vi "niRFSTS SG Close.vi"(11 "TSM Context":T1) -> (0 "error out":errorcluster)   [LabVIEW 2014]
uses:
  <vilib>/NI_TestStand_SemiconductorModule/NI_TestStand_Semiconductor_Module.lvlibp/PinMap/General/SemiconductorModuleContext.ctl
  <vilib>/NI_TestStand_SemiconductorModule/NI_TestStand_Semiconductor_Module.lvlibp/PinMap/RF/RFSG/PinToNIRFSGSessions.vi
  <vilib>/NI_TestStand_SemiconductorModule/NI_TestStand_Semiconductor_Module.lvlibp
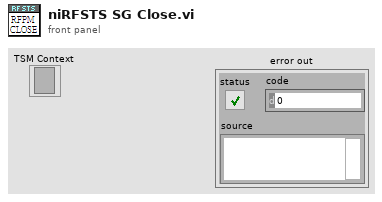
[diagram p1: front panel]
types:
  T1 = typedef "NI_TestStand_Semiconductor_Module.lvlibp/SemiconductorModuleContext.ctl" = refnum<k7>
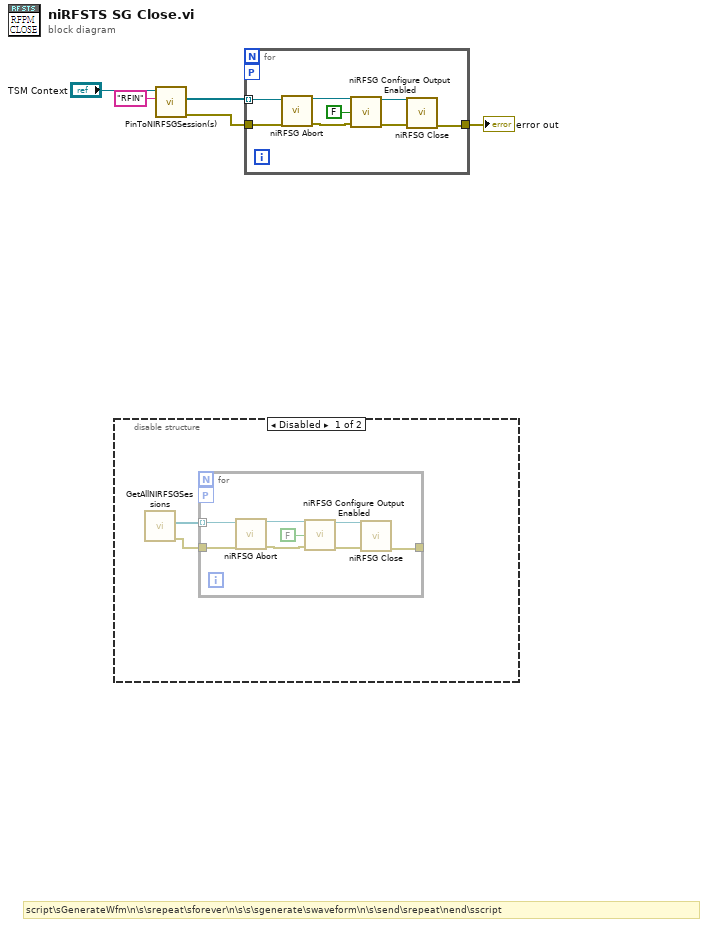
[diagram p0: block diagram]
diagram:
  # "script\\sGenerateWfm\\n\\s\\srepeat\\sforever\\n\\s\\s\\sgenerate\\swaveform\\n\\s\\send\\srepeat\\nend\\sscript"
  n1 = disable-structure shown="Disabled" {
    frame Disabled {
      n2 = call <vilib>:"GetAllNIRFSGSessions.vi"() -> ("error out"=w7:errorcluster, "Instrument Sessions"=w6:refnum<k15>[])  [unwired: 9 in, 1 out]
      n3 = for {
        workers-P: _ -> [_]
        tunnel: w6 -> [w11] mode=indexing
        tunnel: w7 -> [w10]
        tunnel: [w12] -> _
        n4 = call <instrlib>:"niRFSG Abort.vi"("instrument handle"=w11, "error in"=w10) -> ("instrument handle out"=w8:refnum<k15>, "error out"=w9:errorcluster)  [unwired: 12 in]
        n5 = call <instrlib>:"niRFSG Configure Output Enabled.vi"("instrument handle"=w8, "output enabled"=FALSE, "error in"=w9) -> ("instrument handle out"=w15:refnum<k15>, "error out"=w14:errorcluster)  [unwired: 11 in]
        n6 = call <instrlib>:"niRFSG Close.vi"("instrument handle"=w15, "error in"=w14) -> ("error out"=w12:errorcluster)  [unwired: 13 out]
      }
    }
    frame Enabled {
    }
  }
  n7 = call-poly <vilib>:"PinToNIRFSGSession(s).vi"("Pin"="RFIN", "Semiconductor Module Context"="TSM Context") -> ("error out"=w2:errorcluster, "Instrument Sessions"=w3:refnum<k15>[])  [unwired: 6 in, 2 out]
  n8 = for {
    workers-P: _ -> [_]
    tunnel: w3 -> [w19] mode=indexing
    tunnel: w2 -> [w18]
    tunnel: [w20] -> w5
    n9 = call <instrlib>:"niRFSG Abort.vi"("instrument handle"=w19, "error in"=w18) -> ("instrument handle out"=w16:refnum<k15>, "error out"=w17:errorcluster)  [unwired: 12 in]
    n10 = call <instrlib>:"niRFSG Configure Output Enabled.vi"("instrument handle"=w16, "output enabled"=FALSE, "error in"=w17) -> ("instrument handle out"=w23:refnum<k15>, "error out"=w22:errorcluster)  [unwired: 11 in]
    n11 = call <instrlib>:"niRFSG Close.vi"("instrument handle"=w23, "error in"=w22) -> ("error out"=w20:errorcluster)  [unwired: 13 out]
  }
  "error out" <- w5
